vi "Stop Freezer.vi"(8 "error in (no error)":errorcluster, 11 "Heater in":refnum<class "Heater.lvclass">) -> (0 "error out":errorcluster, 3 "Heater out":refnum<class "Heater.lvclass">)   [LabVIEW 2015, in "cRIO-Carbondioxide.lvlib" / "CO2-Actor.lvlib" / "Heater.lvclass"]
uses:
  Heater.lvclass
  Heater.lvclass/Heater.ctl
  <vilib>/ActorFramework/Message Enqueuer/Message Enqueuer.lvclass/Message Enqueuer.ctl
  <vilib>/ActorFramework/Message Enqueuer/Enqueue.vi
  <vilib>/ActorFramework/Message Priority Queue/Priority Enqueue.vi
  <vilib>/ActorFramework/Stop Msg/Stop Msg.lvclass
  CO2 Actor/CO2 Actor.lvclass
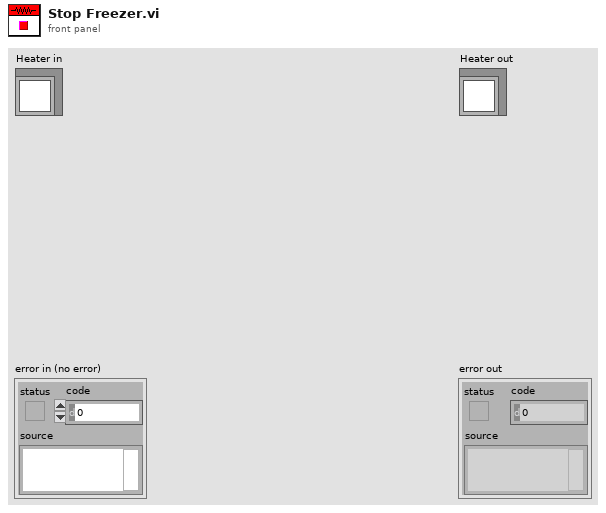
[diagram p1: front panel]
types:
  T1 = typedef "cRIO-Carbondioxide.lvlib/cRIO-CO2.lvlib/cRIO-CO2.lvclass/Freezers Enumerator.ctl" = enum16{"Undefined", "Syringe", "Cold Tank 1", "Cold Tank 2", "Cold Tank 3", "Cold Tank 4"}
  T2 = typedef "Dedicated Enqueuers.ctl" = cluster{"Freezers":cluster{"Syringe":refnum<class "Message Enqueuer.lvclass">, "Tank 1":refnum<class "Message Enqueuer.lvclass">, "Tank 2":refnum<class "Message Enqueuer.lvclass">, "Tank 3":refnum<class "Message Enqueuer.lvclass">, "Tank 4":refnum<class "Message Enqueuer.lvclass">}, "Heaters":cluster{"Syringe":refnum<class "Message Enqueuer.lvclass">, "Piston":refnum<class "Message Enqueuer.lvclass">}, "Blowers":cluster{"Tank 1":refnum<class "Message Enqueuer.lvclass">, "Tank 2":refnum<class "Message Enqueuer.lvclass">, "Tank 3":refnum<class "Message Enqueuer.lvclass">, "Tank 4":refnum<class "Message Enqueuer.lvclass">, "Syringe":refnum<class "Message Enqueuer.lvclass">}, "Sample Line":refnum<class "Message Enqueuer.lvclass">, "Storage Line":refnum<class "Message Enqueuer.lvclass">, "Transfer Line":refnum<class "Message Enqueuer.lvclass">, "Syringe Stepper":refnum<class "Message Enqueuer.lvclass">, "Syringe Line":refnum<class "Message Enqueuer.lvclass">, "Capillary Line":refnum<class "Message Enqueuer.lvclass">, "Preparation Line":refnum<class "Message Enqueuer.lvclass">, "Turbo":refnum<class "Message Enqueuer.lvclass">, "Vacuum":refnum<class "Message Enqueuer.lvclass">, "He Line":refnum<class "Message Enqueuer.lvclass">, "Cylinder":refnum<class "Message Enqueuer.lvclass">}
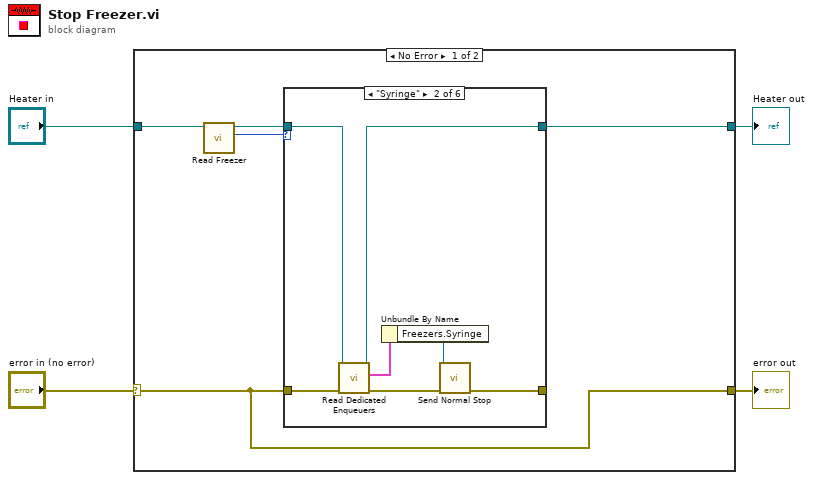
[diagram p0: block diagram]
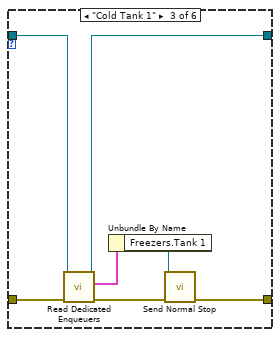
[diagram p3: hidden frame]
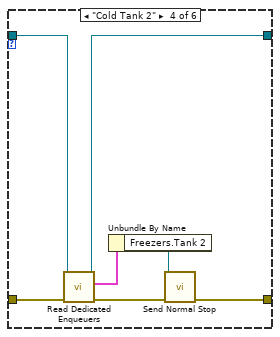
[diagram p4: hidden frame]
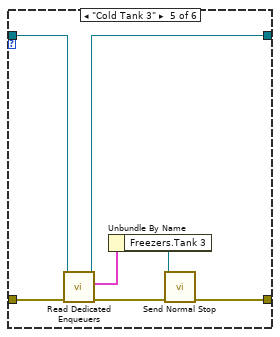
[diagram p5: hidden frame]
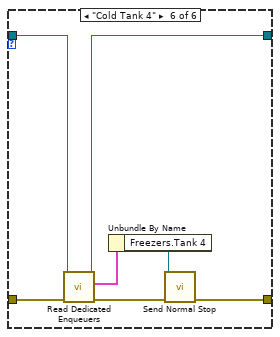
[diagram p6: hidden frame]
diagram:
  n1 = case shown="No Error" "error in (no error)" {
    selector: "error in (no error)" -> [w5 w48]
    tunnel: [w5 w48] -> w3
    tunnel: [w7 w47] -> w1
    tunnel: "Heater in" -> [w9 w47]
    frame No Error {
      n2 = call "Read Freezer.vi"("Heater in"=w9) -> ("Freezer"=w6:T1, "Heater out"=w8:refnum<class "Heater.lvclass">)  [unwired: 9 in]
      n3 = case shown="\"Syringe\"" w6 {
        tunnel: w5 -> [w10 w18 w25 w32 w39 w46]
        tunnel: w8 -> [w11 w17 w24 w31 w38 w45]
        tunnel: [w11 w16 w23 w30 w37 w44] -> w7
        tunnel: [w10 w13 w19 w27 w33 w40] -> _
        frame "Undefined", Default {
        }
        frame "Syringe" {
          n4 = call "Read Dedicated Enqueuers.vi"("error in (no error)"=w18, "CO2 Actor in"=w17) -> ("error out"=w14:errorcluster, "Dedicated Enqueuers"=w15:T2, "CO2 Actor out"=w16:refnum<class "Heater.lvclass">)  [unwired: 6 in, 1 out]
          n5 = Unbundle By Name(w15) -> ("Freezers.Syringe"=w12:refnum<class "Message Enqueuer.lvclass">)
          n6 = call <vilib>:"Send Normal Stop.vi"("error in (no error)"=w14, "Message Enqueuer"=w12) -> ("error out"=w13:errorcluster)  [unwired: 9 in]
        }
        frame "Cold Tank 1" {
          n7 = call "Read Dedicated Enqueuers.vi"("error in (no error)"=w25, "CO2 Actor in"=w24) -> ("error out"=w21:errorcluster, "Dedicated Enqueuers"=w22:T2, "CO2 Actor out"=w23:refnum<class "Heater.lvclass">)  [unwired: 6 in, 1 out]
          n8 = Unbundle By Name(w22) -> ("Freezers.Tank 1"=w20:refnum<class "Message Enqueuer.lvclass">)
          n9 = call <vilib>:"Send Normal Stop.vi"("error in (no error)"=w21, "Message Enqueuer"=w20) -> ("error out"=w19:errorcluster)  [unwired: 9 in]
        }
        frame "Cold Tank 2" {
          n10 = call "Read Dedicated Enqueuers.vi"("error in (no error)"=w32, "CO2 Actor in"=w31) -> ("error out"=w28:errorcluster, "Dedicated Enqueuers"=w29:T2, "CO2 Actor out"=w30:refnum<class "Heater.lvclass">)  [unwired: 6 in, 1 out]
          n11 = Unbundle By Name(w29) -> ("Freezers.Tank 2"=w26:refnum<class "Message Enqueuer.lvclass">)
          n12 = call <vilib>:"Send Normal Stop.vi"("error in (no error)"=w28, "Message Enqueuer"=w26) -> ("error out"=w27:errorcluster)  [unwired: 9 in]
        }
        frame "Cold Tank 3" {
          n13 = call "Read Dedicated Enqueuers.vi"("error in (no error)"=w39, "CO2 Actor in"=w38) -> ("error out"=w35:errorcluster, "Dedicated Enqueuers"=w36:T2, "CO2 Actor out"=w37:refnum<class "Heater.lvclass">)  [unwired: 6 in, 1 out]
          n14 = Unbundle By Name(w36) -> ("Freezers.Tank 3"=w34:refnum<class "Message Enqueuer.lvclass">)
          n15 = call <vilib>:"Send Normal Stop.vi"("error in (no error)"=w35, "Message Enqueuer"=w34) -> ("error out"=w33:errorcluster)  [unwired: 9 in]
        }
        frame "Cold Tank 4" {
          n16 = call "Read Dedicated Enqueuers.vi"("error in (no error)"=w46, "CO2 Actor in"=w45) -> ("error out"=w42:errorcluster, "Dedicated Enqueuers"=w43:T2, "CO2 Actor out"=w44:refnum<class "Heater.lvclass">)  [unwired: 6 in, 1 out]
          n17 = Unbundle By Name(w43) -> ("Freezers.Tank 4"=w41:refnum<class "Message Enqueuer.lvclass">)
          n18 = call <vilib>:"Send Normal Stop.vi"("error in (no error)"=w42, "Message Enqueuer"=w41) -> ("error out"=w40:errorcluster)  [unwired: 9 in]
        }
      }
    }
    frame Error {
    }
  }
  "error out" <- w3
  "Heater out" <- w1
